vi "Test Draw Rectangle ARGB.vi"(8 "error in (no error)":errorcluster, 11 "Test Case In":refnum<class "01_Image.lvclass">) -> (0 "error out":errorcluster, 3 "Test Case Out":refnum<class "01_Image.lvclass">)   [LabVIEW 2020, in "test.lvlib" / "01_Image.lvclass"]
uses:
  01_Image.lvclass
  C:/Program Files (x86)/National Instruments/LabVIEW 2026/vi.lib/Astemes/LUnit/Test Case.lvclass
  image/ARGB Colour.ctl
  common/Image Size (Integer).ctl
  common/Image Point (Integer).ctl
  <vilib>/Astemes/LUnit/Test Case.lvclass/Test Case.ctl
  image/New Image (ARGB Preallocated).vi
  4993e8ee-a06a-463a-9684-69129f64d5ce.vi
  image/New Image (ARGB Preallocated).vi/3321fa97-f432-4e1e-8db9-a0df79aed21b.vi
  image/ARGB Colour to U32 Pixel Value.vi
  image/Draw Rectangle (ARGB).vi/7e6fb015-3761-4366-a0a7-e436eb229083.vi
  image/Draw Image to Picture (ARGB).vi/8cd07b1b-062e-4fe4-9e87-2eb3dc89fe0e.vi
  <vilib>/Astemes/LUnit/Core/LUnit Test Case/Private/Append Pass Result.vi
  <vilib>/Astemes/LUnit/Core/LUnit Test Case/Private/Append Fail Result.vi
  4993e8ee-a06a-463a-9684-69129f64d5ce.vi/9c5d11cd-9439-4240-a1ee-d9baace9c924.vi
  <vilib>/Astemes/LUnit/Core/LUnit Test Case/Private/Run In UI.vi
  <vilib>/Utility/error.llb/Clear Errors.vi
  <vilib>/Utility/error.llb/Error Cluster From Error Code.vi
  image/image.lvlib
  common/common.lvlib
panel:
  out "Picture":picture
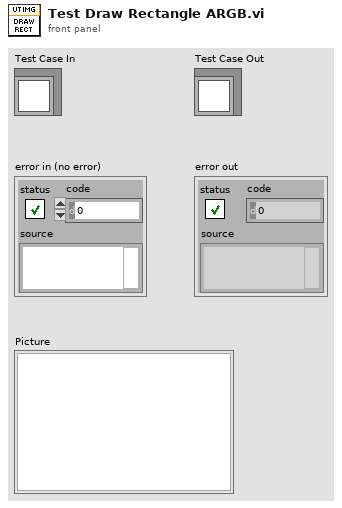
[diagram p1: front panel]
types:
  T1 = typedef "common.lvlib/Image Point (Integer).ctl" = cluster{"x":i32, "y":i32}
  T2 = typedef "image.lvlib/ARGB Colour.ctl" = cluster{"Alpha":u8, "RGB":u32}
  T3 = typedef "common.lvlib/Image Size (Integer).ctl" = cluster{"Width":u16, "Height":u16}
  T4 = typedef "image.lvlib/ARGB Image.ctl" = refnum<data-value>
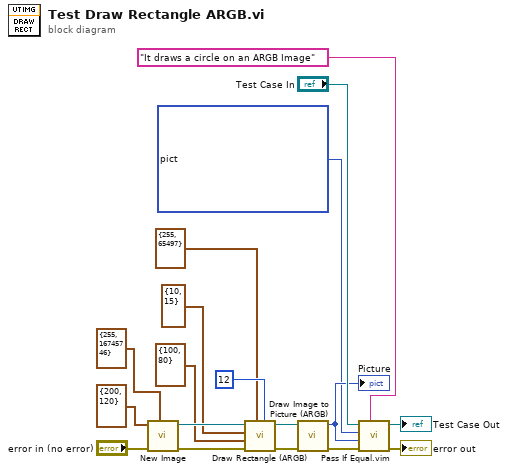
[diagram p0: block diagram]
diagram:
  n1 = call-poly "New Image.vi"("Colour (Default: Black)"=T2 {"Alpha"=255, "RGB"=16745746}, "error in (no error)"="error in (no error)", "Preallocated Image Size (Default: 0,0)"=T3 {"Width"=200, "Height"=120}) -> ("error out"=w11:errorcluster, "ARGB Image"=w12:T4)  [unwired: 7 in]
  n2 = call "Draw Rectangle (ARGB).vi"("Thickness (Default: 1)"=u16 12, "ARGB Colour"=T2 {"Alpha"=255, "RGB"=65497}, "error in (no error)"=w11, "Point B"=T1 {"x"=100, "y"=80}, "Point A"=T1 {"x"=10, "y"=15} ("Centre"), "ARGB Image in"=w12) -> ("error out"=w9:errorcluster, "ARGB Image"=w10:T4)  [unwired: 4 in]
  n3 = call "Draw Image to Picture (ARGB).vi"("error in (no error)"=w9, "ARGB Image Source in"=w10) -> ("error out"=w14:errorcluster, "Picture"=w5:picture)  [unwired: 8 in]
  "Picture" <- w5
  n4 = call "Pass If Equal.vim"("Description"="It draws a circle on an ARGB Image", "error in (no error)"=w14, "Actual"=w5, "Expected"=picture bytes[72030] ("Picture"), "LUnit Test Case In"="Test Case In") -> ("error out"=→"error out":errorcluster, "LUnit Test Case Out"=→"Test Case Out":refnum<class "01_Image.lvclass">)  [unwired: 5 in]
